vi "ma_Locate three fingers (FFT input).vi"(2 "spectrum includes end points?":bool, 3 "criterion":T2 {"Threshold" format="%.2f"}, 4 "spectral info":T1 {"window" items=["Rectangle"=0, "Hanning"=1, "Hamming"=2, "Blackman-Harris"=3, "Exact Blackman"=4, "Blackman"=5, "Flat Top"=6, "4 Term B-Harris "=7, "7 Term B-Harris"=8, "Low Sidelobe"=9, "Blackman Nuttall"=11, "Triangle"=30, "Bartlett-Hanning"=31, "Bohman"=32, "Parzen"=33, "Welch"=34, "Kaiser"=60, "Dolph-Chebyshev"=61, "Gaussian"=62]}, 5 "FFT spectrum":T3={"f0"=0.0, "df"=1.0, "spectrum"=[]} {"spectrum" format="%.2f"; "df" format="%.2f"; "f0" format="%.2f"}) -> (0 "number of tones":i32, 1 "three fingers (frequency normalized)":T3[](array[typedef]) {"spectrum" format="%.2f"; "df" format="%.2f"; "f0" format="%.2f"})   [LabVIEW 2020, in "NI_MAPro.lvlib"]
uses:
  NI_MAPro.lvlib
  ma_sml_Spectrum Cluster (complex).ctl
  ma_sml_Spectral Info.ctl
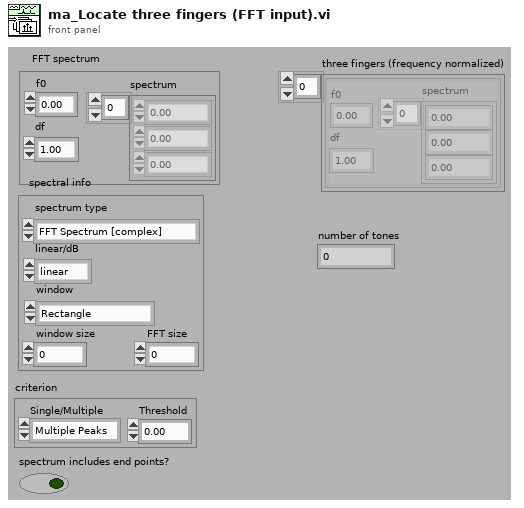
[diagram p1: front panel]
types:
  T1 = typedef "NI_MAPro.lvlib/ma_sml_Spectral Info.ctl" = cluster{"spectrum type":enum16{"FFT Spectrum [complex]", "Amplitude [Magnitude]", "Power [Magnitude^2]", "Cross Spectrum [complex]", "Frequency Response [Complex]"}, "linear/dB":enum16{"linear", "dB"}, "window":u16, "window size":i32, "FFT size":i32}
  T2 = cluster{"Single/Multiple":enum16{"Multiple Peaks", "Single Max Peak"}, "Threshold":dbl}
  T3 = typedef "NI_MAPro.lvlib/ma_sml_Spectrum Cluster (complex).ctl" = cluster{"f0":dbl, "df":dbl, "spectrum":cdb[]}
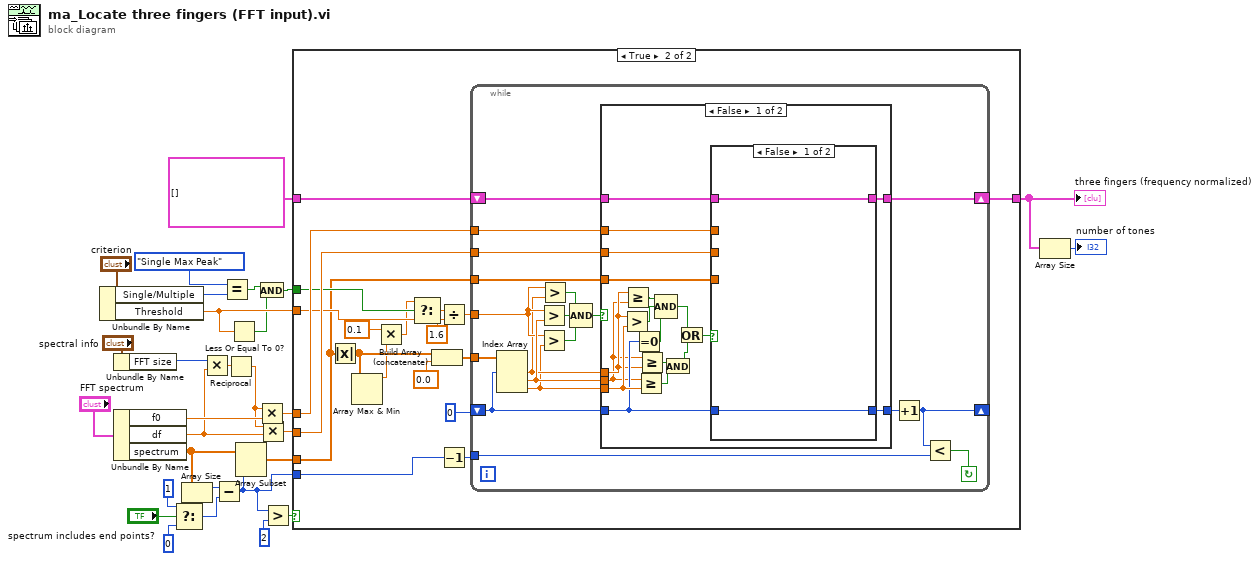
[diagram p0: block diagram]
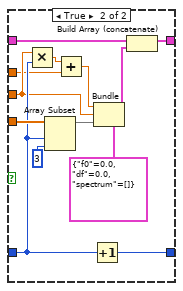
[diagram p3: hidden frame]
diagram:
  n1 = Unbundle By Name("criterion") -> ("Single/Multiple"=w15:enum16{"Multiple Peaks", "Single Max Peak"}, "Threshold"=w4:dbl)
  n2 = Unbundle By Name("spectral info") -> ("FFT size"=w21:i32)
  n3 = Unbundle By Name("FFT spectrum") -> ("f0"=w28:dbl, "df"=w18:dbl, "spectrum"=w6:cdb[])
  n4 = Select(t=1, s="spectrum includes end points?", f=0) -> (s? t:f=w11:i32)
  n5 = Array Size(array=w6) -> (size(s)=w12:i32)
  n6 = Multiply(x=w21, y=w18) -> (x*y=w17:dbl)
  n7 = Subtract(x=w12, y=w11) -> (x-y=w5:i32)
  n8 = Equal?(x=enum16{"Multiple Peaks", "Single Max Peak"}."Single Max Peak" ("Single/Multiple"), y=w15) -> (x = y?=w13:bool)
  n9 = Reciprocal(x=w17) -> (1/x=w16:dbl)
  n10 = Less Or Equal To 0?(x=w4) -> (x <= 0?=w2:bool)
  n11 = Array Subset(array=w6, length=w5) -> (w7:cdb[])  [unwired: 1 in]
  n12 = And(x=w13, y=w2) -> (x .and. y?=w3:bool)
  n13 = Multiply(x=w16, y=w28) -> (x*y=w20:dbl)
  n14 = Multiply(x=w16, y=w18) -> (x*y=w19:dbl)
  n15 = Greater?(x=w5, y=2) -> (0:w27:bool)
  n16 = case shown="True" w27 {
    tunnel: w4 -> [_ w40]
    tunnel: w20 -> [_ w49]
    tunnel: w19 -> [_ w48]
    tunnel: [w30 w47] -> w24
    tunnel: w7 -> [_ w35]
    tunnel: T3[] [] ("three fingers (frequency normalized)") -> [w30 w46]
    tunnel: w3 -> [_ w41]
    tunnel: w5 -> [_ w34]
    frame False {
    }
    frame True {
      n17 = Absolute Value(x=w35) -> (abs(x)=w39:dbl[])
      n18 = Array Max & Min(array=w39) -> (max value=w38:dbl)  [unwired: 3 out]
      n19 = Multiply(x=0.1, y=w38) -> (x*y=w36:dbl)
      n20 = Select(t=w36, s=w41, f=w40) -> (s? t:f=w32:dbl)
      n21 = Build Array (concatenate)(w39, 0.0 ("df")) -> (w44:dbl[])
      n22 = Divide(x=w32, y=1.6) -> (x/y=w33:dbl)
      n23 = Decrement(x=w34) -> (x-1=w42:i32)
      n24 = while {
        tunnel: w42 -> [w57]
        tunnel: w48 -> [w61]
        tunnel: w49 -> [w62]
        tunnel: w35 -> [w63]
        shift-left: w46 -> [w64]
        shift-right: [w60] -> w47
        tunnel: w33 -> [w55]
        shift-left: 0 -> [w66]
        shift-right: [w58] -> _
        tunnel: w44 -> [w68]
        stop <- w59 continue-if-true
        n25 = Index Array(array=w68, index #1=w66) -> (element #1=w54:dbl, element #2=w56:dbl, element #3=w53:dbl)  [unwired: 2 in]
        n26 = Greater?(x=w55, y=w56) -> (0:w67:bool)
        n27 = Greater?(x=w55, y=w53) -> (0:w50:bool)
        n28 = Greater?(x=w55, y=w54) -> (0:w51:bool)
        n29 = Compound Arithmetic op=AND(w51, w67, w50) -> (w52:bool)
        n30 = case shown="False" w52 {
          tunnel: [w84 w103] -> w65
          tunnel: w66 -> [w74 w103]
          tunnel: w53 -> [w78 _]
          tunnel: w54 -> [w70 _]
          tunnel: w64 -> [w83 w102]
          tunnel: w63 -> [w82 _]
          tunnel: w62 -> [w81 _]
          tunnel: w61 -> [w80 _]
          tunnel: [w79 w102] -> w60
          tunnel: w56 -> [w69 _]
          frame False {
            n31 = Greater?(x=w70, y=w78) -> (0:w76:bool)
            n32 = Greater Or Equal?(x=w70, y=w69) -> (x >= y?=w77:bool)
            n33 = Equal To 0?(x=w74) -> (x = 0?=w75:bool)
            n34 = Greater Or Equal?(x=w69, y=w78) -> (x >= y?=w85:bool)
            n35 = Greater Or Equal?(x=w69, y=w70) -> (x >= y?=w86:bool)
            n36 = Compound Arithmetic op=AND(w77, w76, w75) -> (w71:bool)
            n37 = And(x=w86, y=w85) -> (x .and. y?=w73:bool)
            n38 = Or(x=w71, y=w73) -> (x .or. y?=w72:bool)
            n39 = case shown="False" w72 {
              tunnel: w74 -> [w88 w99]
              tunnel: [w88 w101] -> w84
              tunnel: w83 -> [w87 w92]
              tunnel: w82 -> [_ w100]
              tunnel: w81 -> [_ w94]
              tunnel: w80 -> [_ w96]
              tunnel: [w87 w90] -> w79
              frame False {
              }
              frame True {
                n40 = Multiply(x=w96, y=w99) -> (x*y=w95:dbl)
                n41 = Array Subset(array=w100, index=w99, length=3 ("Array Length")) -> (w97:cdb[])
                n42 = Add(x=w95, y=w94) -> (x+y=w93:dbl)
                n43 = Increment(x=w99) -> (x+1=w101:i32)
                n44 = Bundle(cluster=T3 {"f0"=0.0, "df"=0.0, "spectrum"=[]} ("FFT spectrum 2"), "f0"=w93, "df"=w96, "spectrum"=w97) -> (w91:T3)
                n45 = Build Array (concatenate)(w92, w91) -> (w90:T3[])
              }
            }
          }
          frame True {
          }
        }
        n46 = Increment(x=w65) -> (x+1=w58:i32)
        n47 = Less?(x=w58, y=w57) -> (x < y?=w59:bool)
      }
    }
  }
  "three fingers (frequency normalized)" <- w24
  n48 = Array Size(array=w24) -> (size(s)=→"number of tones":i32)
